vi "Write Horsepower.vi"(8 "error in (no error)":errorcluster, 10 "Horsepower":i32, 11 "Car in":refnum<class "Car.lvclass">) -> (0 "error out":errorcluster, 3 "Car out":refnum<class "Car.lvclass">)   [LabVIEW 2019, in "Car.lvclass"]
uses:
  Car.lvclass
  Car.lvclass/Car.ctl
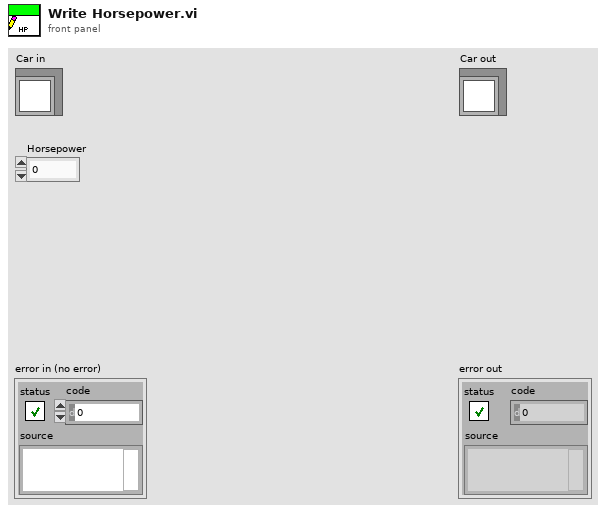
[diagram p1: front panel]
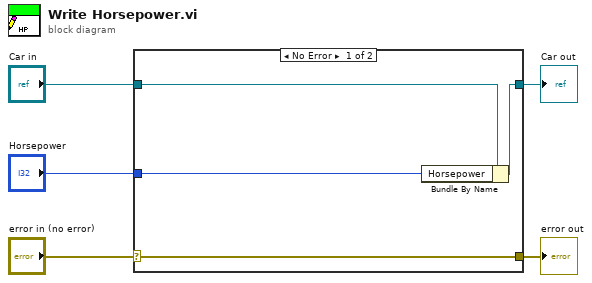
[diagram p0: block diagram]
diagram:
  n1 = case shown="No Error" "error in (no error)" {
    selector: "error in (no error)" -> [w9 w10]
    tunnel: [w9 w10] -> w4
    tunnel: [w7 w11] -> w2
    tunnel: "Car in" -> [w8 w11]
    tunnel: "Horsepower" -> [w6 _]
    frame No Error {
      n2 = Bundle By Name(cluster=w8, "Horsepower"=w6) -> (w7:refnum<class "Car.lvclass">)
    }
    frame Error {
    }
  }
  "error out" <- w4
  "Car out" <- w2
